vi "Show ROI for Pattern.vi"(8 "error in (no error)":errorcluster, 9 "Vision tool":string, 10 "Image":T1(plugin-control), 11 "multi coloum list box":string[][](array[string])) -> (0 "error out":errorcluster, 1 "Pattern Rsult":T2(array[cluster]), 3 "Image 3":T1(plugin-control))   [LabVIEW 2020]
uses:
  <vilib>/vision/NI_Vision_Development_Module.lvlib
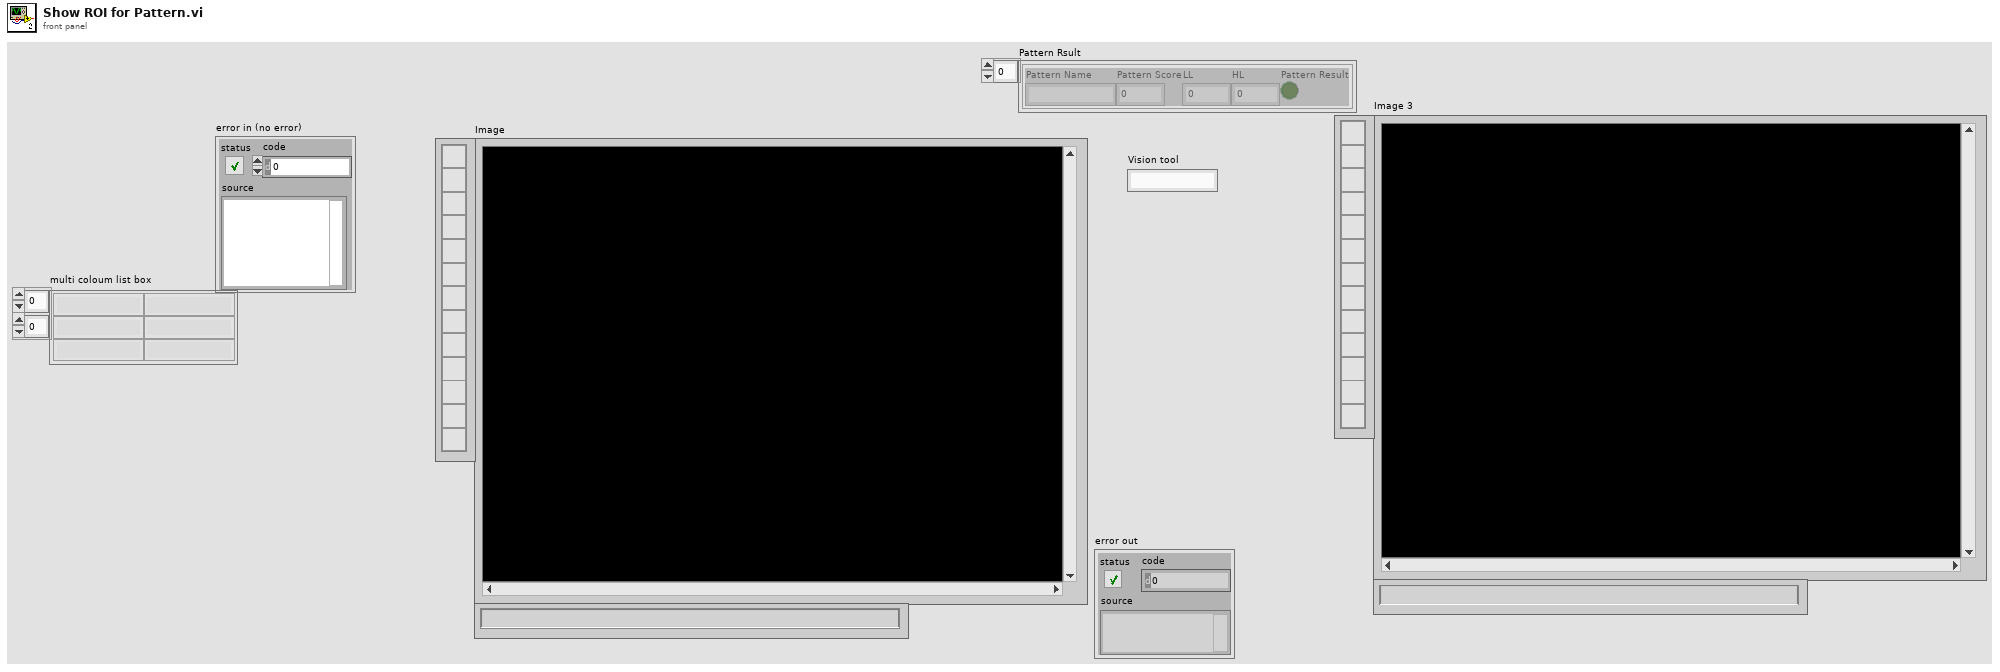
[diagram p1: front panel]
types:
  T1 = typedef "IMAQ Image.ctl" = refnum<image>
  T2 = cluster{"Pattern Name":string, "Pattern Score":dbl, "LL":dbl, "HL":dbl, "Pattern Result":bool}[]
  T3 = cluster{"Pattern Name":string, "Pattern Score":dbl, "LL":dbl, "HL":dbl, "Pattern Result":bool}
  T4 = cluster{"Global Rectangle":i32[], "Contours":cluster{"Contour Type":u32, "ROI Type":u32, "Points":i32[]}[]}
  T5 = typedef "Image Type" = u32
  T6 = typedef "ROI Descriptor" = cluster{"Global Rectangle":i32[], "Contours":cluster{"ID":enum32{"External", "Internal"}, "Type":u32, "Coordinates":i32[]}[]}
  T7 = cluster{"Position":cluster{"x":sgl, "y":sgl}, "Angle":sgl, "Scale":sgl, "Score":sgl, "Bounding Box":cluster{"x":sgl, "y":sgl}[]}[]
  T8 = cluster{"Position":cluster{"x":sgl, "y":sgl}, "Angle":sgl, "Scale":sgl, "Score":sgl, "Bounding Box":cluster{"x":sgl, "y":sgl}[]}
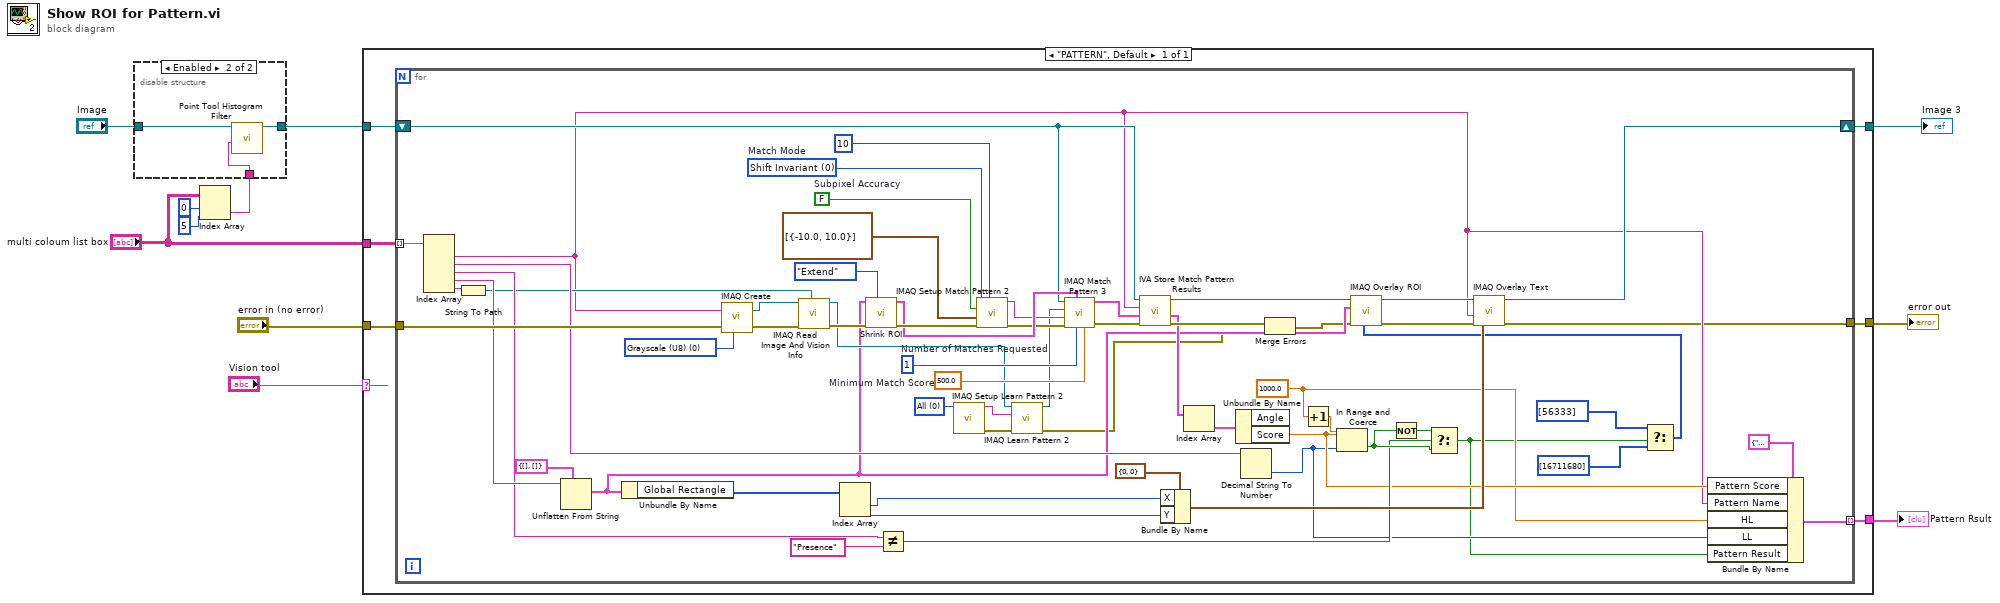
[diagram p0: block diagram]
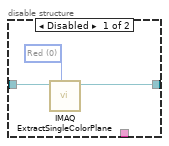
[diagram p2: hidden frame]
diagram:
  n1 = Index Array(array="multi coloum list box", index (row)=0, index (col)=5 ("disabled index (col)")) -> (element=w1:string)
  n2 = disable-structure shown="Enabled" {
    disable-tunnel: "Image" -> [w12 w17]
    disable-tunnel: [w14 w16] -> w5
    disable-tunnel: w1 -> [_ w15]
    frame Disabled {
      w13 = 0 items=["Red", "Green", "Blue", "Hue", "Saturation", "Luminance", "Value", "Intensity"] ("Color Plane")
      n3 = call "IMAQ ExtractSingleColorPlane"("Color Plane"=w13, "Image Src"=w12) -> ("Image Dst Out"=w14:T1)  [unwired: 2 in, 7 out]
    }
    frame Enabled {
      n4 = call "Point Tool Histogram Filter.vi"("Combo Box"=w15, "Image in"=w17) -> ("Image out"=w16:T1)  [unwired: 8 in, 1 out]
    }
  }
  n5 = case shown="\"PATTERN\", Default" "Vision tool" {
    tunnel: "error in (no error)" -> [w23]
    tunnel: w5 -> [w22]
    tunnel: "multi coloum list box" -> [w21]
    tunnel: [w20] -> w10
    tunnel: [w19] -> w9
    tunnel: [w18] -> w8
    frame "PATTERN", Default {
      n6 = for {
        tunnel: w23 -> [w72]
        tunnel: w21 -> [w68] mode=indexing
        shift-right: [w41] -> w18
        shift-left: w22 -> [w64]
        tunnel: [w39] -> w20 mode=indexing
        tunnel: [w33] -> w19
        w30 = u16 0 items=["All", "Shift Information", "Rotation Information"] ("Learn Mode")
        w37 = 1000.0 ("HL")
        w66 = sgl 500.0  # Minimum Match Score
        w67 = 1  # Number of Matches Requested
        w75 = FALSE  # Subpixel Accuracy
        w76 = u16 0 items=["Shift Invariant", "Rotation Invariant"]  # Match Mode
        w71 = T5 0 items=["Grayscale (U8)", "Grayscale (I16)", "Grayscale (SGL)", "Complex (CSG)", "RGB (U32)", "HSL (U32)", "RGB (U64)", "Grayscale (U16)"] ("Image Type")
        n7 = Index Array(array=w68) -> (element #1=w34:string, element #2=w61:string, element #3=w48:string, element #4=w51:string, element #5=w43:string)  [unwired: 5 in]
        n8 = String To Path(string=w43) -> (path=w42:path)
        n9 = Unflatten From String(type=T4 {"Global Rectangle"=[], "Contours"=[]} ("ROI"), binary string=w51) -> (value=w26:T4)  [unwired: 3 in, 2 out]
        n10 = Unbundle By Name(w26) -> ("Global Rectangle"=w58:i32[])
        n11 = call "IMAQ Create"("Image Name"=w34, "Image Type"=w71, "error in (no error)"=w72) -> ("New Image"=w84:T1, "error out"=w70:errorcluster)  [unwired: 2 in]
        n12 = call "IMAQ Read Image And Vision Info"("File Path"=w42, "error in (no error)"=w70, "Image"=w84) -> ("error out"=w80:errorcluster, "Image Out"=w29:T1)  [unwired: 6 in, 1 out]
        n13 = Index Array(array=w58) -> (element #1=w57:i32, element #2=w56:i32)  [unwired: 2 in]
        n14 = call "Shrink ROI.vi"("ROI Change"=enum16{"Extend", "Shrink"}."Extend", "error in (no error)"=w80, "ROI in"=w26) -> ("error out"=w81:errorcluster, "ROI Descriptor"=w79:T6)  [unwired: 7 in]
        n15 = Not Equal?(x=w48, y="Presence") -> (x != y?=w46:bool)
        n16 = call "IMAQ Setup Learn Pattern 2"("Learn Mode"=w30) -> ("error out"=w32:errorcluster, "Learn Pattern Setup Data"=w31:string)  [unwired: 9 in]
        n17 = call "IMAQ Setup Match Pattern 2"("Minimum Contrast"=10, "error in (no error)"=w81, "Rotation Angle Ranges (degrees)"=cluster{sgl, sgl}[] [{-10.0, 10.0}], "Subpixel Accuracy"=w75, "Match Mode"=w76) -> ("error out"=w77:errorcluster, "Match Pattern Setup Data"=w74:string)  [unwired: 5 in]
        n18 = call "IMAQ Learn Pattern 2"("error in (no error)"=w32, "Learn Pattern Setup Data"=w31, "Image"=w29) -> ("error out"=w24:errorcluster, "Template Image Out"=w28:T1)  [unwired: 7 in]
        n19 = call "IMAQ Match Pattern 3"("Minimum Match Score"=w66, "Number of Matches Requested"=w67, "ROI Descriptor"=w79, "error in (no error)"=w77, "Match Pattern Setup Data"=w74, "Template Image"=w28, "Image"=w64) -> ("error out"=w82:errorcluster, "Matches"=w65:T7)  [unwired: 2 in, 1 out]
        n20 = call <vilib>:"IVA Store Match Pattern Results.vi"("error in (no error)"=w82, "Matches"=w65, "Step Name"=w34, "Image in"=w64) -> ("error out"=w83:errorcluster, "Calibrated Matches"=w62:T7, "Image dup"=w85:T1)  [unwired: 5 out]
        n21 = Bundle By Name(cluster=cluster{"X":i32, "Y":i32} {"X"=0, "Y"=0} ("Origin"), "X"=w57, "Y"=w56) -> (w55:cluster{"X":i32, "Y":i32})
        n22 = Index Array(array=w62) -> (element=w63:T8)  [unwired: 1 in]
        n23 = Unbundle By Name(w63) -> ("Score"=w38:sgl)  [unwired: 1 out]
        n24 = Decimal String To Number(string=w61) -> (number=w36:i32)  [unwired: 2 in, 1 out]
        n25 = Merge Errors(w83, w24) -> (w25:errorcluster)
        n26 = Increment(x=w37) -> (x+1=w59:dbl)
        n27 = In Range and Coerce(upper limit=w59, x=w38, lower limit=w36) -> (In Range?=w47:bool)  [unwired: 1 out]
        n28 = Not(x=w47) -> (.not. x?=w50:bool)
        n29 = Select(t=w50, s=w46, f=w47) -> (s? t:f=w35:bool)
        n30 = Select(t=u32[] [56333] ("Colors (Green)"), s=w35, f=u32[] [16711680] ("Colors (Green)")) -> (s? t:f=w45:u32[])
        n31 = call "IMAQ Overlay ROI"("Colors (Green)"=w45, "error in (no error)"=w25, "ROI Descriptor"=w26, "Image"=w85) -> ("error out"=w54:errorcluster, "Image Out"=w44:T1)  [unwired: 6 in]
        n32 = call "IMAQ Overlay Text"("error in (no error)"=w54, "String"=w34, "Origin"=w55, "Image"=w44) -> ("error out"=w33:errorcluster, "Image Out"=w41:T1)  [unwired: 6 in]
        n33 = Bundle By Name(cluster=T3 {"Pattern Name"="", "Pattern Score"=0.0, "LL"=0.0, "HL"=0.0, "Pattern Result"=FALSE} ("Pattern Single Result"), "Pattern Score"=w38, "Pattern Name"=w34, "HL"=w37, "LL"=w36, "Pattern Result"=w35) -> (w39:T3)
      }
    }
  }
  "Pattern Rsult" <- w10
  "error out" <- w9
  "Image 3" <- w8
